vi "Read PubDataEvents.vi"(11 "UserEvents in":refnum<class "UserEvents.lvclass">) -> (2 "PubDataEvents":T1, 3 "UserEvents out":refnum<class "UserEvents.lvclass">)   [LabVIEW 2013, in "UserEvents.lvclass"]
uses:
  UserEvents.lvclass
  Typedefs/PubDataEvents.ctl
  Typedefs/StateSelector.ctl
  Typedefs/OutputData.ctl
  Typedefs/InputData.ctl
  <userlib>/Common/ILC/Typedefs/ADCs.ctl
  Typedefs/TestStatus.ctl
  Typedefs/TemperatureSettling.ctl
  Typedefs/WaitTimeStatus.ctl
  UserEvents.lvclass/UserEvents.ctl
  Typedefs/AITDTTypedefs.lvlib
  <userlib>/Common/ILC/Typedefs/ILCTypedefs.lvlib
panel:
  # "ADCs"
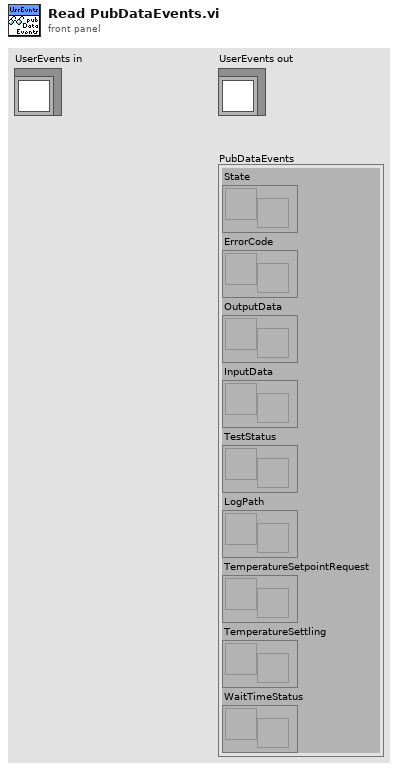
[diagram p1: front panel]
types:
  T1 = typedef "AITDTTypedefs.lvlib/PubDataEvents.ctl" = cluster{"State":refnum<user-event>, "ErrorCode":refnum<user-event>, "OutputData":refnum<user-event>, "InputData":refnum<user-event>, "TestStatus":refnum<user-event>, "LogPath":refnum<user-event>, "TemperatureSetpointRequest":refnum<user-event>, "TemperatureSettling":refnum<user-event>, "WaitTimeStatus":refnum<user-event>}
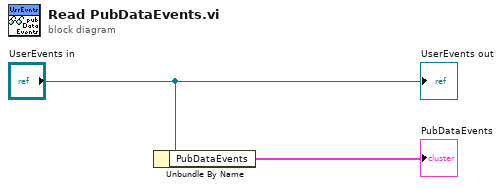
[diagram p0: block diagram]
diagram:
  n1 = Unbundle By Name("UserEvents in") -> ("PubDataEvents"=→"PubDataEvents":T1)
  "UserEvents out" <- "UserEvents in"
